vi "Anti_deadband_FB_PVG.vi"(1 "x":sgl) -> (0 "y":sgl)   [LabVIEW 2017]
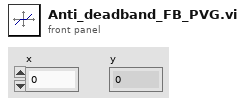
[diagram p1: front panel]
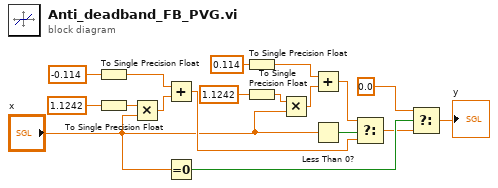
[diagram p0: block diagram]
diagram:
  n1 = To Single Precision Float(number=-0.114 ("t")) -> (single precision float=w7:sgl)
  n2 = To Single Precision Float(number=1.1242 ("t")) -> (single precision float=w15:sgl)
  n3 = Multiply(x=w15, y="x") -> (x*y=w18:sgl)
  n4 = Add(x=w7, y=w18) -> (x+y=w2:sgl)
  n5 = Equal To 0?(x="x") -> (x = 0?=w12:bool)
  n6 = To Single Precision Float(number=0.114 ("t")) -> (single precision float=w9:sgl)
  n7 = To Single Precision Float(number=1.1242 ("t")) -> (single precision float=w17:sgl)
  n8 = Multiply(x=w17, y="x") -> (x*y=w4:sgl)
  n9 = Add(x=w9, y=w4) -> (x+y=w3:sgl)
  n10 = Less Than 0?(x="x") -> (x < 0?=w5:bool)
  n11 = Select(t=w3, s=w5, f=w2) -> (s? t:f=w10:sgl)
  n12 = Select(t=sgl 0.0, s=w12, f=w10) -> (s? t:f=→"y":sgl)
